vi "LJM_eWriteName Example.vi"() -> (0 "error out":errorcluster)   [LabVIEW 2020]
panel:
  out "Error String":string
  in  "Value":dbl=2.5 format="%.6f"
  in  "Name":string="DAC0"
  out "ConnectionType Out":i32
  out "DeviceType Out":i32
  in  "Identifier":string="LJM_idANY"
  in  "ConnectionType":string="LJM_ctANY"
  in  "DeviceType":string="LJM_dtANY"
  # "Common Registers:\nAddress, Name, Type, Read/Write\n0, AIN0, 3, RO\n2, AIN1, 3, RO\n1000, DAC0, 3, RW\n1002, DAC1, 3, RW\n2000, FIO0, 0, RW\n2001, FIO1, 0, RW\n55110, TEST_UINT16, 0, RW\n60000, PRODUCT_ID, 3, RO\n60004, FIRMWARE_VERSION, 3, RO\n60028, SERIAL_NUMBER, 1, RO\n\nTypes: 0=UINT16, 1=UINT32, 2=INT32, 3=FLOAT32"
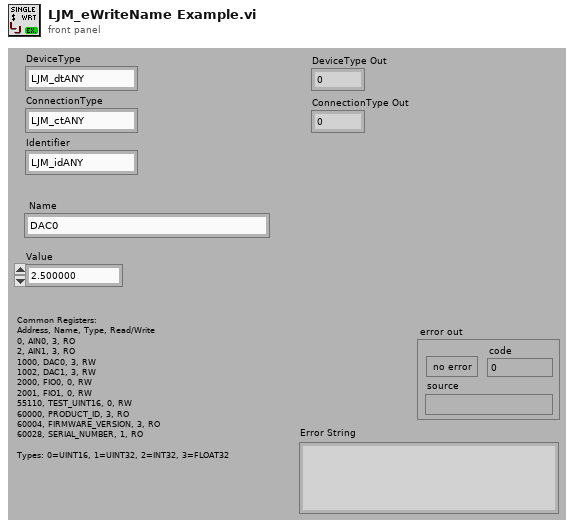
[diagram p1: front panel]
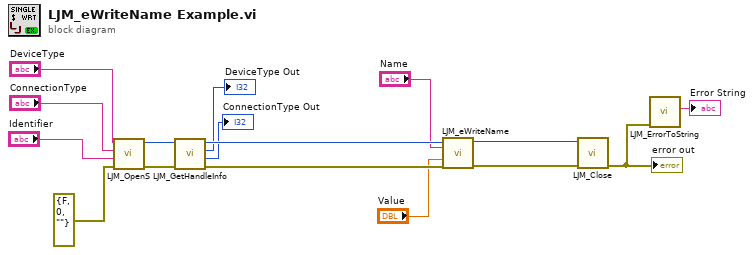
[diagram p0: block diagram]
diagram:
  n1 = call "LJM_OpenS.vi"("error in"=errorcluster {"status"=FALSE, "code"=0, "source"=""} ("error in (no error)"), "Identifier"="Identifier", "ConnectionType"="ConnectionType", "DeviceType"="DeviceType") -> ("error out"=w14:errorcluster, "Handle"=w12:i32)  [unwired: 6 in]
  n2 = call "LJM_GetHandleInfo.vi"("error in"=w14, "Handle In"=w12) -> ("error out"=w13:errorcluster, "ConnectionType"=→"ConnectionType Out":i32, "DeviceType"=→"DeviceType Out":i32, "Handle Out"=w11:i32)  [unwired: 2 in, 4 out]
  n3 = call "LJM_eWriteName.vi"("Handle In"=w11, "Name"="Name", "Value"="Value", "error in"=w13) -> ("Handle Out"=w10:i32, "error out"=w15:errorcluster)  [unwired: 10 in]
  n4 = call "LJM_Close.vi"("error in"=w15, "Handle"=w10) -> ("error out"=w3:errorcluster)  [unwired: 9 in]
  "error out" <- w3
  n5 = call "LJM_ErrorToString.vi"("error in"=w3) -> ("String"=→"Error String":string)  [unwired: 10 in]
